vi "SetSerializableData.vi"(7 "BlueSerializer in":refnum<class "BlueSerializer.lvclass">, 8 "error in (no error)":errorcluster, 10 "Data in":T1={"StructuredData"=variant(string ""), "ClassOps (child, parent)"=[]}, 11 "Golf Player":refnum<class "Golf Player.lvclass">) -> (0 "error out":errorcluster, 2 "Data out":T1={"StructuredData"=variant(string ""), "ClassOps (child, parent)"=[]}, 3 "Golf Player":refnum<class "Golf Player.lvclass">, 5 "BlueSerializer out":refnum<class "BlueSerializer.lvclass">)   [LabVIEW 2020, in "Golf Player.lvclass"]
doc: "Dynamic Dispatch setter to set SerializableData for all inheritance levels of a <b>BlueSerializable</b> class. This and all overrides should ONLY be consumed by a child of <b>SerializerBase</b>"
uses:
  Golf Player.lvclass
  <userlib>/Blue Origin/BlueSerialization/BlueSerializer/BlueSerializer.lvclass
  Sports Player/Sports Player.lvclass
  <userlib>/Blue Origin/BlueSerialization/BlueSerializable/BlueSerializable.lvclass
  <userlib>/Blue Origin/BlueSerialization/BlueSerializer/Support/SetSerializableDataCluster.ctl
  <userlib>/Blue Origin/BlueSerialization/BlueSerializer/Support/SetSerializableDataClusterLayer.ctl
  <userlib>/Blue Origin/BlueSerialization/BlueSerializer/Support/SetSerializableDataClusterIterable.ctl
  <userlib>/Blue Origin/BlueSerialization/BlueSerializer/BlueSerializableVersion.ctl
  <userlib>/Blue Origin/BlueSerialization/BlueSerializer/Support/SetSerializableDataObject.ctl
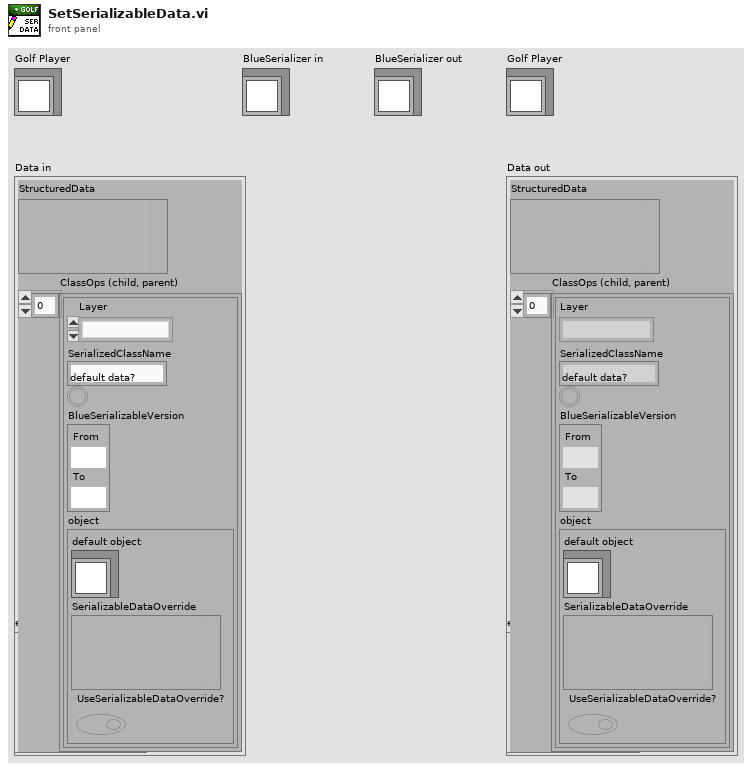
[diagram p1: front panel]
types:
  T1 = typedef "BlueSerialization.lvlib/BlueSerializer.lvclass/SetSerializableDataCluster.ctl" = cluster{"StructuredData":variant, "ClassOps (child, parent)":T2[]}
  T2 = typedef "BlueSerialization.lvlib/BlueSerializer.lvclass/SetSerializableDataClusterIterable.ctl" = cluster{"Layer":T3, "SerializedClassName":string, "default data?":bool, "BlueSerializableVersion":T4, "object":T5}
  T3 = typedef "BlueSerialization.lvlib/BlueSerializer.lvclass/SetSerializableDataClusterLayer.ctl" = enum16{"new class layer", "dropped class layer", "agreed class layer"}
  T4 = typedef "BlueSerialization.lvlib/BlueSerializer.lvclass/BlueSerializableVersion.ctl" = cluster{"From":u16, "To":u16}
  T5 = typedef "BlueSerialization.lvlib/BlueSerializer.lvclass/SetSerializableDataObject.ctl" = cluster{"default object":refnum<class "BlueSerializable.lvclass">, "SerializableDataOverride":variant, "UseSerializableDataOverride?":bool}
  T6 = typedef "Golf Player.lvclass/SerializableData.ctl" = cluster{"League":string, "# holes in one":i32, "longest drive (ft)":dbl}
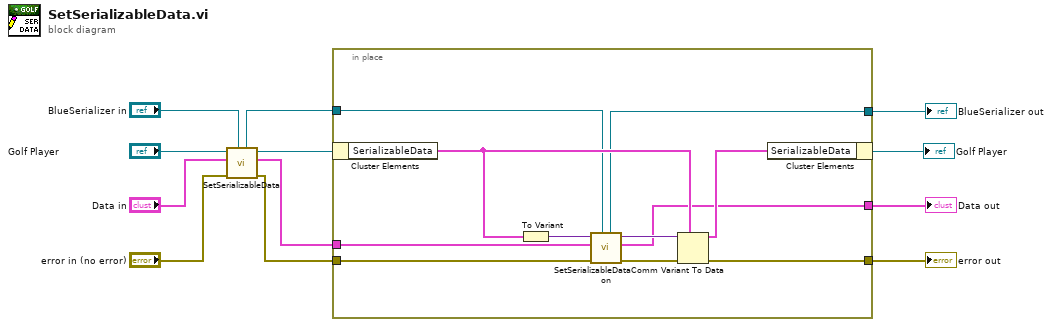
[diagram p0: block diagram]
diagram:
  n1 = call-parent "SetSerializableData.vi"("BlueSerializer in"="BlueSerializer in", "error in (no error)"="error in (no error)", "Data in"="Data in", "Sports Player"="Golf Player") -> ("error out"=w3:errorcluster, "Data out"=w1:T1, "Sports Player"=w4:refnum<class "Golf Player.lvclass">, "BlueSerializer out"=w2:refnum<class "BlueSerializer.lvclass">)  [unwired: 4 in]
  n2 = in-place {
    in-place-border: w3 -> [w22]
    in-place-border: w2 -> [w17]
    in-place-border: [w16] -> w7
    in-place-border: [w15] -> w6
    in-place-border: [w14] -> w5
    in-place-border: w1 -> [w13]
    n3 = in-place-cluster #1(w4) -> ("SerializableData"=w19:T6)
    n4 = To Variant(anything=w19) -> (Variant=w23:variant)
    n5 = call <userlib>:"SetSerializableDataCommon.vi"("BlueSerializer in"=w17, "error in (no error)"=w22, "Data In"=w13, "SerializableData"=w23) -> ("error out"=w21:errorcluster, "Data Out"=w14:T1, "SerializableData"=w20:variant, "BlueSerializer out"=w16:refnum<class "BlueSerializer.lvclass">)  [unwired: 4 in]
    n6 = Variant To Data(error in=w21, type=w19, Variant=w20) -> (data=w18:T6, error out=w15:errorcluster)
    n7 = in-place-cluster #1("SerializableData"=w18) -> (→"Golf Player":refnum<class "Golf Player.lvclass">)
  }
  "error out" <- w6
  "Data out" <- w5
  "BlueSerializer out" <- w7
